vi "GetIntegrationTime.vi"(8 "error in":errorcluster {"code" format="%.0x"}, 10 "ArgIndex(0)":i32, 11 "Args":string[](array[string])) -> (0 "error out":errorcluster {"code" format="%.0x"}, 2 "ExposureTime(mSec)":string, 3 "ExposureTime(Sec)":dbl)   [LabVIEW 2020]
doc: "Retreive the exposure time from the 'Args' array"
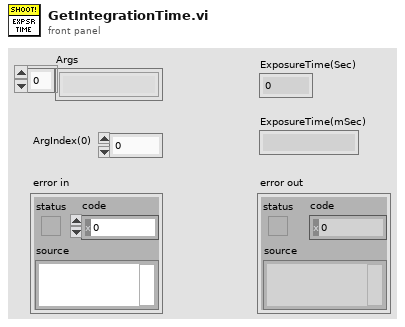
[diagram p1: front panel]
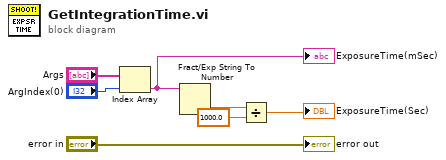
[diagram p0: block diagram]
diagram:
  n1 = Index Array(array="Args", index="ArgIndex(0)") -> (element=w3:string)
  "ExposureTime(mSec)" <- w3
  n2 = Fract/Exp String To Number(string=w3) -> (number=w4:dbl)  [unwired: 3 in, 1 out]
  n3 = Divide(x=w4, y=1000.0) -> (x/y=→"ExposureTime(Sec)":dbl)
  "error out" <- "error in"
